vi "Get package_template_enum for Value.vi"(8 "error in (no error)":errorcluster, 10 "value in proto":i32, 11 "gRPC ID":T1) -> (0 "error out":errorcluster, 2 "value in LV":u32, 3 "gRPC ID Out":T1)   [LabVIEW 2019, in "Service Template.lvlib"]
uses:
  Service Template.lvlib
  <vilib>/gRPC/LabVIEW gRPC Library/Shared/grpcId.ctl
  <vilib>/Utility/error.llb/Error Cluster From Error Code.vi
  <vilib>/Utility/error.llb/Simple Error Handler.vi
  <vilib>/gRPC/LabVIEW gRPC Library/grpc-lvsupport-release.lvlib
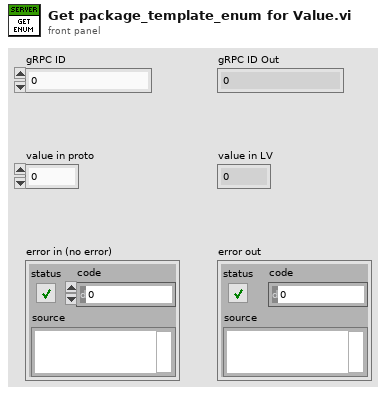
[diagram p1: front panel]
types:
  T1 = typedef "grpc-lvsupport-release.lvlib/grpcId.ctl" = u64
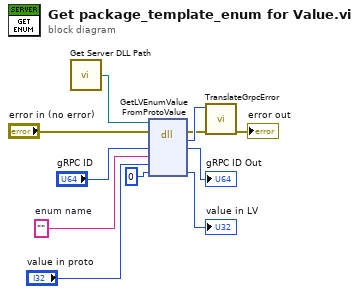
[diagram p0: block diagram]
diagram:
  w10 = ""  # enum name
  n1 = call <vilib>:"Get Server DLL Path.vi"() -> ("Server dll path"=w1:path)
  n2 = dll-call lib="?" fn="GetLVEnumValueFromProtoValue"(path in=w1, error in="error in (no error)", "gRPC ID in"="gRPC ID", "enum name"=w10, "value in proto"="value in proto", "value in LV"=u32 0) -> (error out=w4:errorcluster, "error code"=w5:i32, "gRPC ID in"=→"gRPC ID Out":T1, "value in LV"=→"value in LV":u32)  [unwired: 3 in, 1 out]
  n3 = call <vilib>:"TranslateGrpcError.vi"("error in"=w4, "Error Code"=w5) -> ("error out"=→"error out":errorcluster)  [unwired: 9 in]
